vi "sub vi - check network dir v1.vi"(11 "PATH":path) -> (0 "error":bool)   [LabVIEW 2013]
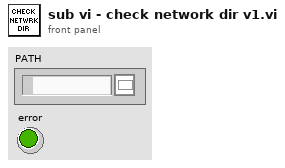
[diagram p1: front panel]
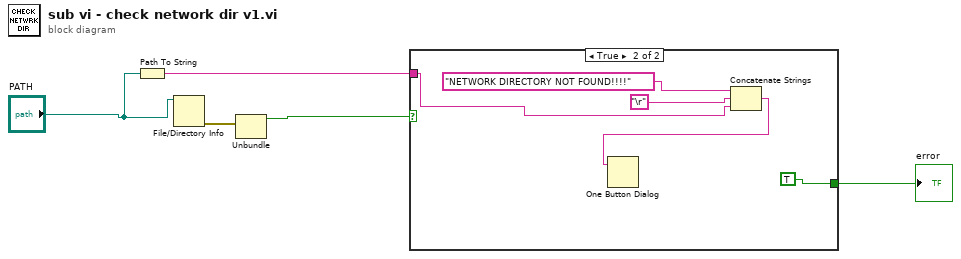
[diagram p0: block diagram]
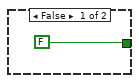
[diagram p2: hidden frame]
diagram:
  n1 = Path To String(path="PATH") -> (string=w5:string)
  n2 = File/Directory Info(path="PATH") -> (error out=w3:errorcluster)  [unwired: 1 in, 6 out]
  n3 = Unbundle(w3) -> ("status"=w4:bool)  [unwired: 2 out]
  n4 = case shown="True" w4 {
    tunnel: w5 -> [_ w9]
    tunnel: [FALSE TRUE] -> w2
    frame False {
    }
    frame True {
      n5 = Concatenate Strings("NETWORK DIRECTORY NOT FOUND!!!!", "\r", w9) -> (w8:string)
      n6 = One Button Dialog(message=w8) -> ()  [unwired: 1 in, 1 out]
    }
  }
  "error" <- w2
